vi "RenderLine.vi"(4 "Y2":sgl, 6 "X2":sgl, 8 "No Error":errorcluster, 9 "Y1":sgl, 10 "X1":sgl, 11 "Renderer [SDL_Renderer *]":i64) -> (0 "error out":errorcluster)   [LabVIEW 2024, in "SDL3.lvlib" / "Render.lvlib"]
doc: "<B>Summary</B>\nDraw a line on the current rendering target at subpixel precision.\n\n<B>Thread Safety</B>\nYou may only call this function from the main thread."
uses:
  Render.lvlib
  Error/Error.lvlib
  Lib/SDL3-32.dll
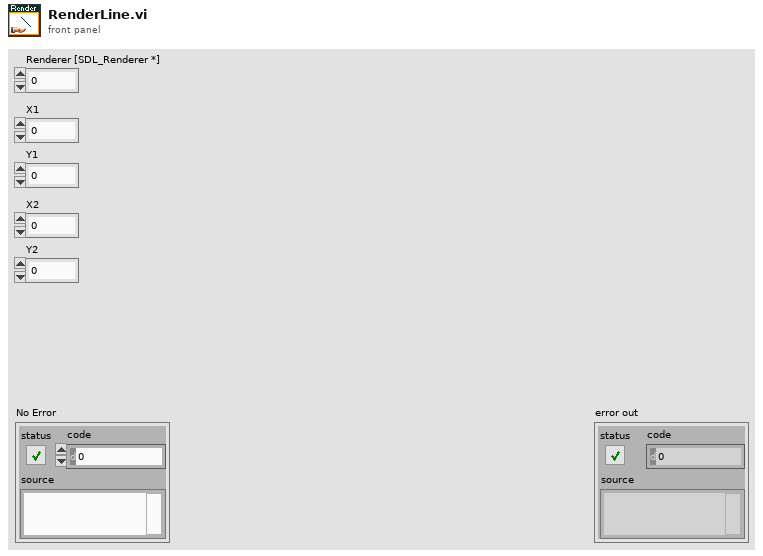
[diagram p1: front panel]
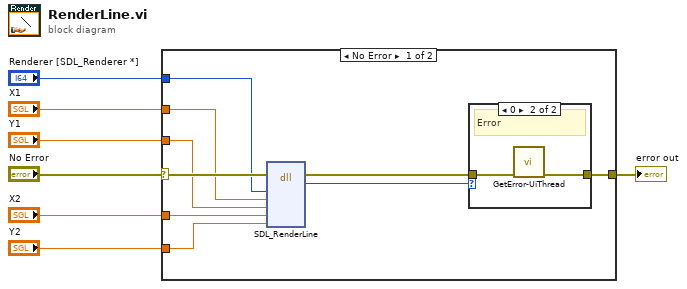
[diagram p0: block diagram]
diagram:
  n1 = case shown="No Error" "No Error" {
    selector: "No Error" -> [w16 w20]
    tunnel: [w14 w20] -> w6
    tunnel: "Renderer [SDL_Renderer *]" -> [w12 _]
    tunnel: "X1" -> [w11 _]
    tunnel: "Y1" -> [w10 _]
    tunnel: "X2" -> [w9 _]
    tunnel: "Y2" -> [w8 _]
    frame No Error {
      n2 = dll-call lib="C:/Users/Thomas/Documents/Projects/LV-SDL3/Lib/SDL3-*.*" fn="SDL_RenderLine"(error in=w16, "renderer"=w12, "x1"=w11, "y1"=w10, "x2"=w9, "y2"=w8) -> (error out=w15:errorcluster, "return type"=w13:i32)  [unwired: 7 in, 1 out]
      n3 = case shown="0" w13 {
        tunnel: w15 -> [w17 w19]
        tunnel: [w17 w18] -> w14
        frame Default {
          # "Ok"
        }
        frame 0 {
          # "Error"
          n4 = call "GetError-UiThread.vi"("No Error"=w19) -> ("error out"=w18:errorcluster)  [unwired: 10 in]
        }
      }
    }
    frame Error {
    }
  }
  "error out" <- w6
